vi "Export JUnit.vi"() -> (3 "FAILURE CAPTURED IN REPORT":bool)   [LabVIEW 2013]
uses:
  classes/Test Suite/Test Suite.lvclass
  classes/Test Suite/Define Test Suite (JUnit Report).vi
  classes/Assert/Assert Greater Or Equal_Variant.vi
  classes/Test/Test.lvclass
  classes/Assert/Assert.lvclass
panel:
  out "Test Report File Contents":string
  out "error out":errorcluster
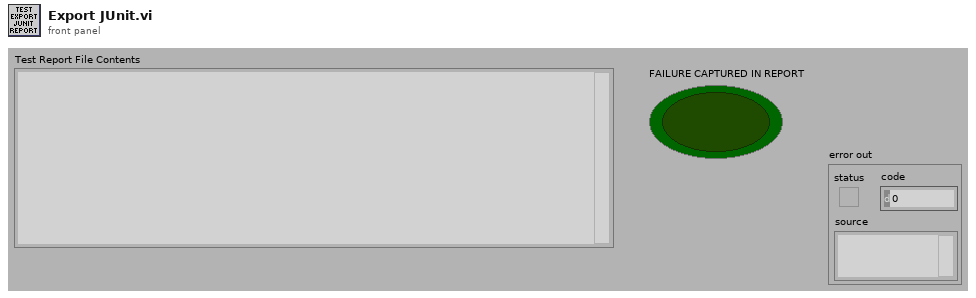
[diagram p1: front panel]
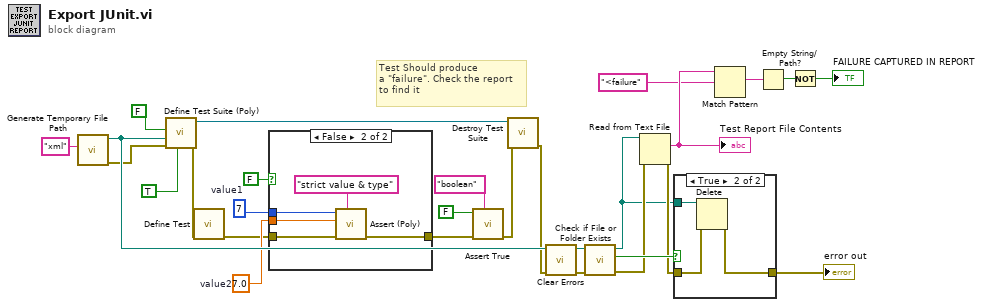
[diagram p0: block diagram]
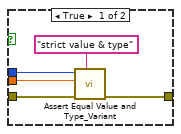
[diagram p2: hidden frame]
diagram:
  w4 = 7.0  # value2
  w5 = 7  # value1
  # "Test Should produce\na \"failure\". Check the report\nto find it"
  n1 = call <vilib>:"Generate Temporary File Path.vi"("Temporary File Extension (tmp)"="xml") -> ("error out"=w18:errorcluster, "Unique Temporary File Path"=w19:path)  [unwired: 9 in]
  n2 = call-poly "Define Test Suite (Poly).vi"("Verbose (F)"=TRUE, "error in (no error)"=w18, "Report Path"=w19, "Interactive"=FALSE) -> ("error out"=w16:errorcluster, "Test Suite"=w27:refnum<class "Test Suite.lvclass">)  [unwired: 6 in]
  n3 = call "Define Test.vi"("error in (no error)"=w16) -> ("error out"=w3:errorcluster)  [unwired: 10 in]
  n4 = case shown="False" FALSE {
    tunnel: w5 -> [w31 w35]
    tunnel: w4 -> [w30 w34]
    tunnel: w3 -> [w29 w37]
    tunnel: [w28 w36] -> w2
    frame True {
      n5 = call "Assert Equal Value and Type_Variant.vi"("Label"="strict value & type", "error in (no error)"=w29, "Y"=w30, "X"=w31) -> ("error out"=w28:errorcluster)  [unwired: 7 in]
    }
    frame False {
      n6 = call-poly "Assert (Poly).vi"("Label"="strict value & type", "error in (no error)"=w37, "Y"=w34, "X"=w35) -> ("error out"=w36:errorcluster)  [unwired: 7 in]
    }
  }
  n7 = call "Assert True.vi"("Label"="boolean", "error in (no error)"=w2, "True?"=FALSE) -> ("error out"=w7:errorcluster)  [unwired: 8 in]
  n8 = call-dynamic "Destroy Test Suite.vi"("error in (no error)"=w7, "Test Suite in"=w27) -> ("error out"=w15:errorcluster)  [unwired: 9 in]
  n9 = call <vilib>:"Clear Errors.vi"("error in (no error)"=w15) -> ("error out"=w14:errorcluster)  [unwired: 6 in]
  n10 = call <vilib>:"Check if File or Folder Exists.vi"("error in (no error)"=w14, "path"=w19) -> ("error out"=w23:errorcluster, "file or folder exists?"=w24:bool, "dup path"=w21:path)  [unwired: 7 in]
  n11 = Read from Text File(file (use dialog)=w21, error in=w23) -> (text=w13:string, error out=w22:errorcluster)  [unwired: 2 in, 2 out]
  "Test Report File Contents" <- w13
  n12 = case shown="True" w24 {
    tunnel: w21 -> [_ w41]
    tunnel: w22 -> [w38 w40]
    tunnel: [w38 w39] -> w17
    frame False {
    }
    frame True {
      n13 = Delete(path (use dialog)=w41, error in=w40) -> (error out=w39:errorcluster)  [unwired: 3 in, 2 out]
    }
  }
  "error out" <- w17
  n14 = Match Pattern(string=w13, regular expression="<failure") -> (match substring=w11:string)  [unwired: 1 in, 3 out]
  n15 = Empty String/Path?(string/path=w11) -> (empty?=w10:bool)
  n16 = Not(x=w10) -> (.not. x?=→"FAILURE CAPTURED IN REPORT":bool)
